vi "Number03to2bitarr.vi"(1 "Value 0-3":i32) -> (0 "2 bit array":bool[](array[boolean]))   [LabVIEW 2017]
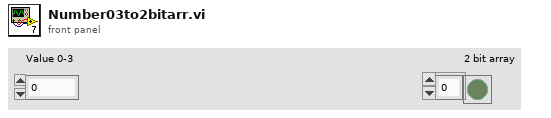
[diagram p1: front panel]
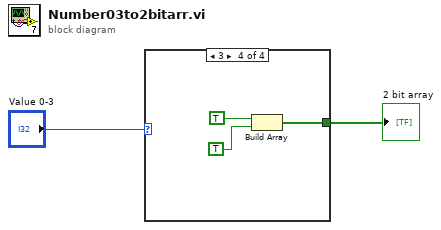
[diagram p0: block diagram]
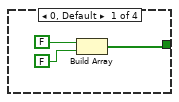
[diagram p2: hidden frame]
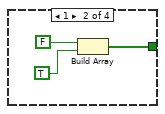
[diagram p3: hidden frame]
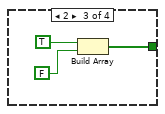
[diagram p4: hidden frame]
diagram:
  n1 = case shown="3" "Value 0-3" {
    tunnel: [w3 w6 w9 w12] -> w2
    frame 0, Default {
      n2 = Build Array(FALSE, FALSE) -> (w3:bool[])
    }
    frame 1 {
      n3 = Build Array(FALSE, TRUE) -> (w6:bool[])
    }
    frame 2 {
      n4 = Build Array(TRUE, FALSE) -> (w9:bool[])
    }
    frame 3 {
      n5 = Build Array(TRUE, TRUE) -> (w12:bool[])
    }
  }
  "2 bit array" <- w2
